vi "Bezahlen.vi"(8 "error in (no error)":errorcluster, 10 "Pries":dbl) -> (0 "error out":errorcluster, 2 "Betrag erreiht":bool)   [LabVIEW 2023]
panel:
  out "Restgeldausgabe":dbl
  in  "Storno":bool
  out "Guthaben":dbl
  in  "100 Euro":bool
  in  "50 Euro":bool
  in  "20 Euro":bool
  in  "10 Euro":bool
  in  "5 Euro":bool
  in  "2 Euro":bool
  in  "Bezahlen":bool
  in  "1 Euro":bool
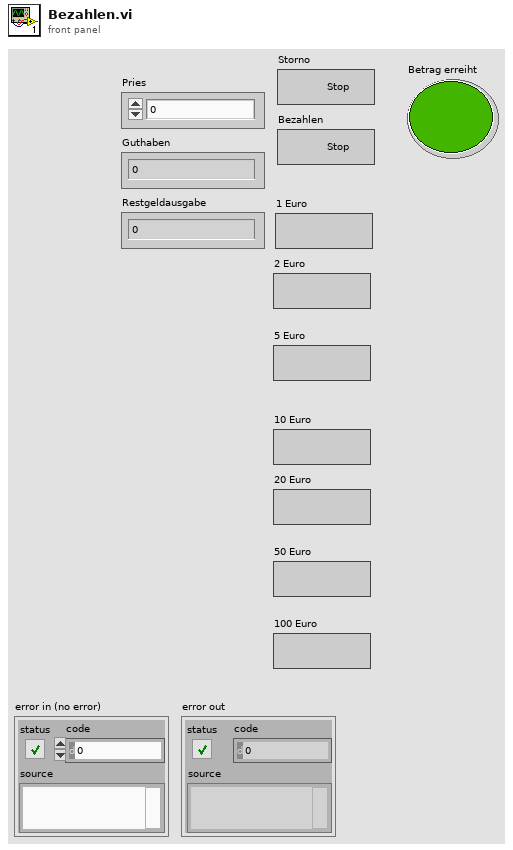
[diagram p1: front panel]
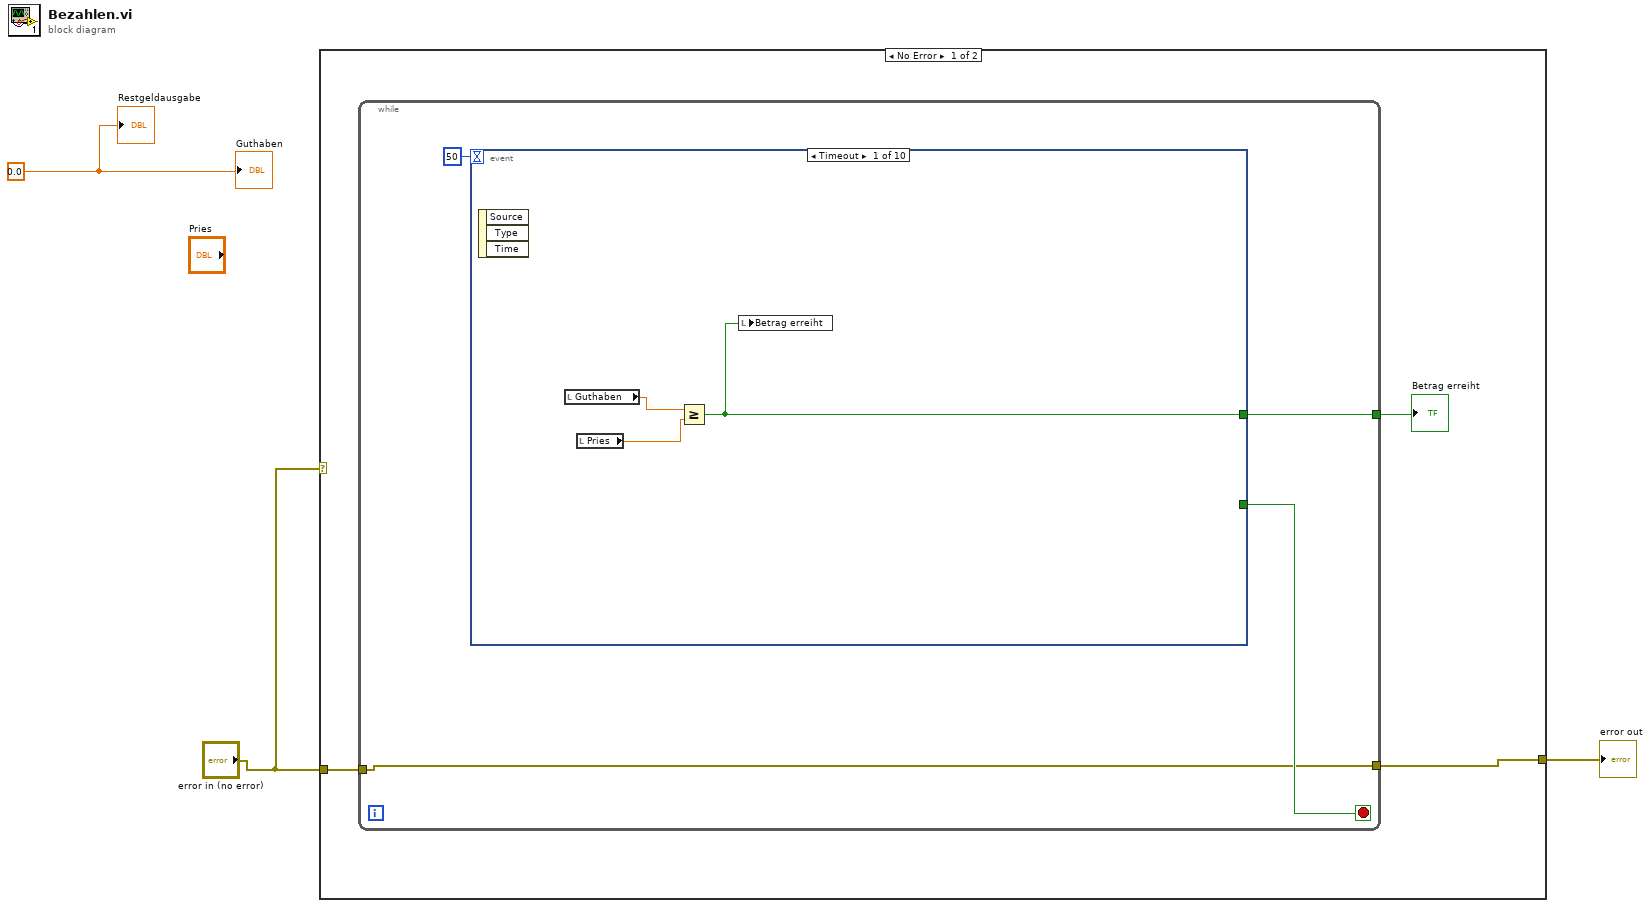
[diagram p0: block diagram]
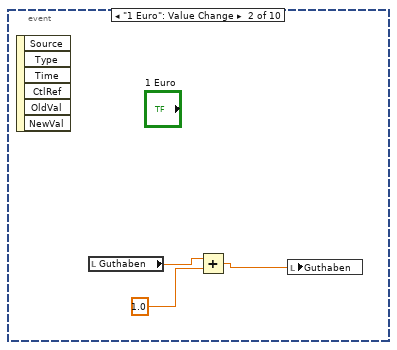
[diagram p2: hidden frame]
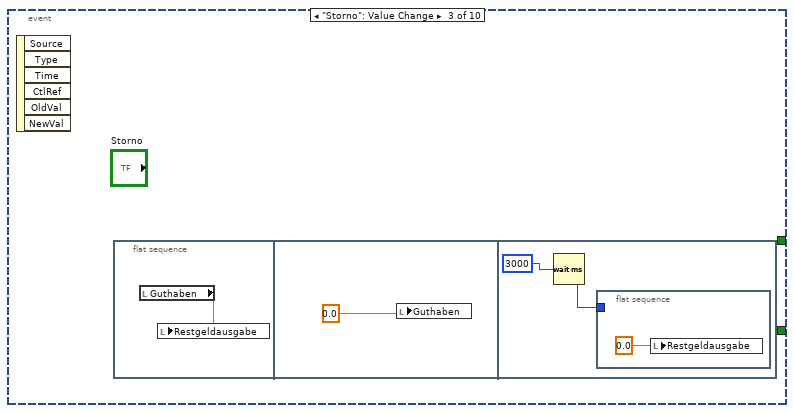
[diagram p3: hidden frame]
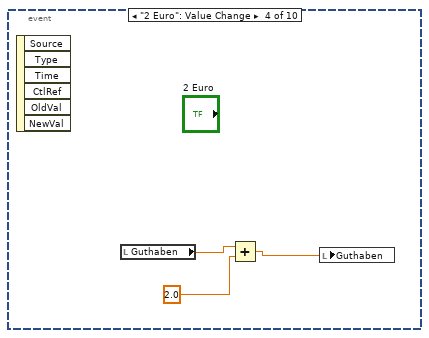
[diagram p4: hidden frame]
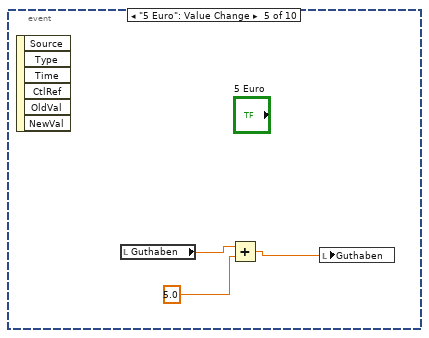
[diagram p5: hidden frame]
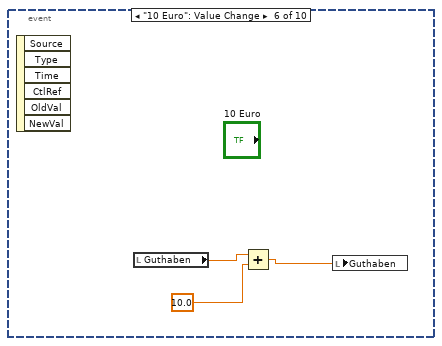
[diagram p6: hidden frame]
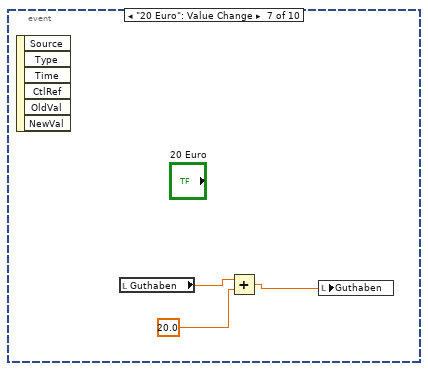
[diagram p7: hidden frame]
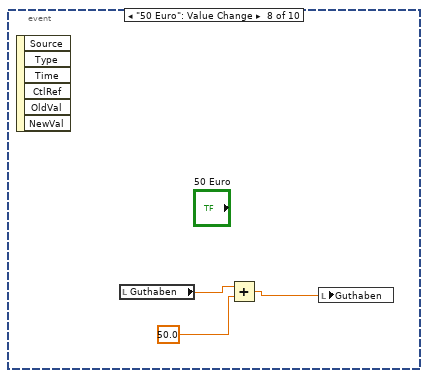
[diagram p8: hidden frame]
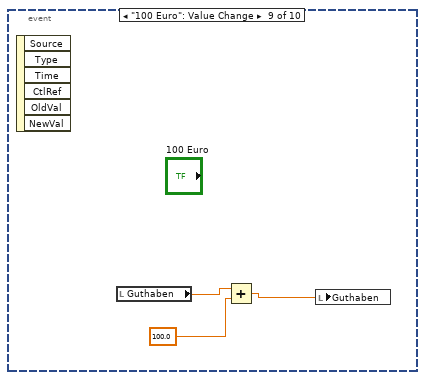
[diagram p9: hidden frame]
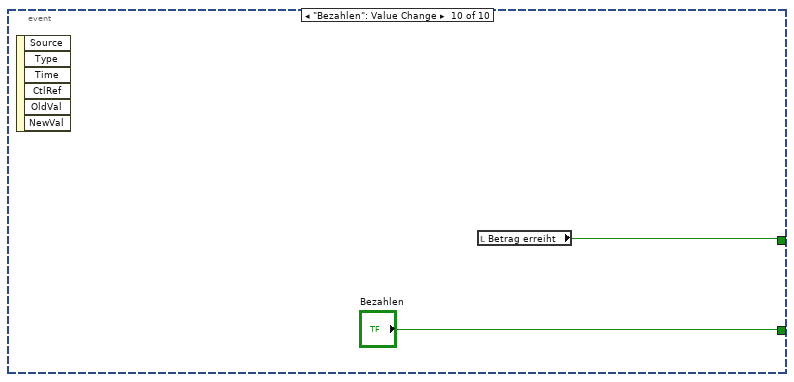
[diagram p10: hidden frame]
diagram:
  w3 = 0.0 ("Guthaben")
  n1 = case shown="No Error" "error in (no error)" {
    tunnel: "error in (no error)" -> [w5 w42]
    tunnel: [w4 w42] -> w2
    frame No Error {
      n2 = while {
        tunnel: [w9] -> w6
        tunnel: w5 -> [w8]
        tunnel: [w8] -> w4
        stop <- w10 stop-if-true
        n3 = event shown="[0] Timeout" {
          selector: _ -> [_ _ _ _ _ _ _ _ _ _]
          dyn-events: _ -> [_ _ _ _ _ _ _ _ _ _]
          timeout: 50 -> [_ _ _ _ _ _ _ _ _ _]
          tunnel: [_ _ _ _ _ _ _ _ _ "Bezahlen"] -> w10
          tunnel: [w11 _ _ _ _ _ _ _ _ w40] -> w9
          event Timeout {
            n4 = event-data() -> ()  [unwired: 1 in, 3 out]
            n5 = local read "Guthaben"() -> (w13:dbl)
            n6 = local read "Pries"() -> (w12:dbl)
            n7 = Greater Or Equal?(x=w13, y=w12) -> (x >= y?=w11:bool)
            n8 = local write "Betrag erreiht"(w11) -> ()
          }
          event "1 Euro": Value Change {
            n9 = event-data() -> ()  [unwired: 1 in, 6 out]
            n10 = local read "Guthaben"() -> (w16:dbl)
            n11 = Add(x=w16, y=1.0) -> (x+y=w14:dbl)
            n12 = local write "Guthaben"(w14) -> ()
          }
          event "Storno": Value Change {
            n13 = event-data() -> ()  [unwired: 1 in, 6 out]
            n14 = flat-sequence {
              frame #0 {
                n15 = local read "Guthaben"() -> (w17:dbl)
                n16 = local write "Restgeldausgabe"(w17) -> ()
              }
              frame #1 {
                n17 = local write "Guthaben"(0.0 ("Guthaben")) -> ()
              }
              frame #2 {
                n18 = Wait (ms)(milliseconds to wait=u32 3000) -> (millisecond timer value=w19:u32)
                n19 = flat-sequence {
                  tunnel: w19 -> [_]
                  frame #0 {
                    n20 = local write "Restgeldausgabe"(0.0 ("Restgeldausgabe")) -> ()
                  }
                }
              }
            }
          }
          event "2 Euro": Value Change {
            n21 = event-data() -> ()  [unwired: 1 in, 6 out]
            n22 = local read "Guthaben"() -> (w24:dbl)
            n23 = Add(x=w24, y=2.0) -> (x+y=w23:dbl)
            n24 = local write "Guthaben"(w23) -> ()
          }
          event "5 Euro": Value Change {
            n25 = event-data() -> ()  [unwired: 1 in, 6 out]
            n26 = local read "Guthaben"() -> (w27:dbl)
            n27 = Add(x=w27, y=5.0) -> (x+y=w26:dbl)
            n28 = local write "Guthaben"(w26) -> ()
          }
          event "10 Euro": Value Change {
            n29 = event-data() -> ()  [unwired: 1 in, 6 out]
            n30 = local read "Guthaben"() -> (w30:dbl)
            n31 = Add(x=w30, y=10.0) -> (x+y=w29:dbl)
            n32 = local write "Guthaben"(w29) -> ()
          }
          event "20 Euro": Value Change {
            n33 = event-data() -> ()  [unwired: 1 in, 6 out]
            n34 = local read "Guthaben"() -> (w33:dbl)
            n35 = Add(x=w33, y=20.0) -> (x+y=w32:dbl)
            n36 = local write "Guthaben"(w32) -> ()
          }
          event "50 Euro": Value Change {
            n37 = event-data() -> ()  [unwired: 1 in, 6 out]
            n38 = local read "Guthaben"() -> (w36:dbl)
            n39 = Add(x=w36, y=50.0) -> (x+y=w35:dbl)
            n40 = local write "Guthaben"(w35) -> ()
          }
          event "100 Euro": Value Change {
            n41 = event-data() -> ()  [unwired: 1 in, 6 out]
            n42 = local read "Guthaben"() -> (w39:dbl)
            n43 = Add(x=w39, y=100.0) -> (x+y=w38:dbl)
            n44 = local write "Guthaben"(w38) -> ()
          }
          event "Bezahlen": Value Change {
            n45 = event-data() -> ()  [unwired: 1 in, 6 out]
            n46 = local read "Betrag erreiht"() -> (w40:bool)
          }
        }
      }
      "Betrag erreiht" <- w6
    }
    frame Error {
    }
  }
  "error out" <- w2
  "Guthaben" <- w3
  "Restgeldausgabe" <- w3
